vi "OpenDevice.vi"(9 "pIdentifier":i64, 10 "mode":i32, 11 "error in (no error)":errorcluster) -> (1 "return type":i32, 2 "hDev":i64, 3 "error out":errorcluster)   [LabVIEW 2016]
uses:
  MVSDKmd.dll
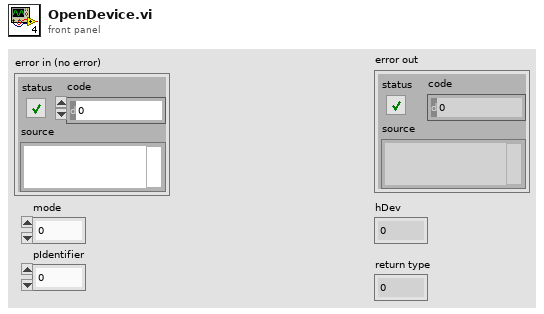
[diagram p1: front panel]
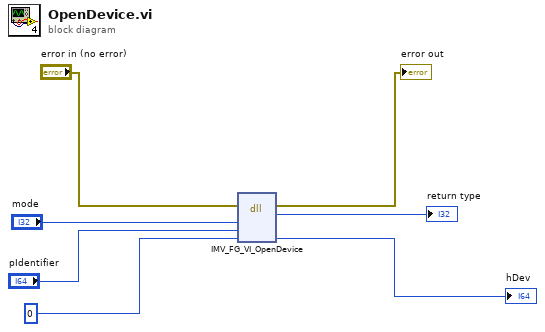
[diagram p0: block diagram]
diagram:
  n1 = dll-call lib="MVSDKmd.dll" fn="IMV_FG_VI_OpenDevice"(error in="error in (no error)", "mode"="mode", "pIdentifier"="pIdentifier", "hDev"=i64 0) -> (error out=→"error out":errorcluster, "return type"=→"return type":i32, "hDev"=→"hDev":i64)  [unwired: 4 in, 1 out]
